vi "CLD 8 CSV file commands utility Exercise.vi"(8 "Error In":errorcluster) -> (0 "Error Out":errorcluster, 3 "Commands Out Array":T1[](array[typedef]))   [LabVIEW 2018]
doc: "CLD 8 exercise"
uses:
  CLD 8 Data Cluster.ctl
  <vilib>/Utility/file.llb/Read Delimited Spreadsheet (string).vi
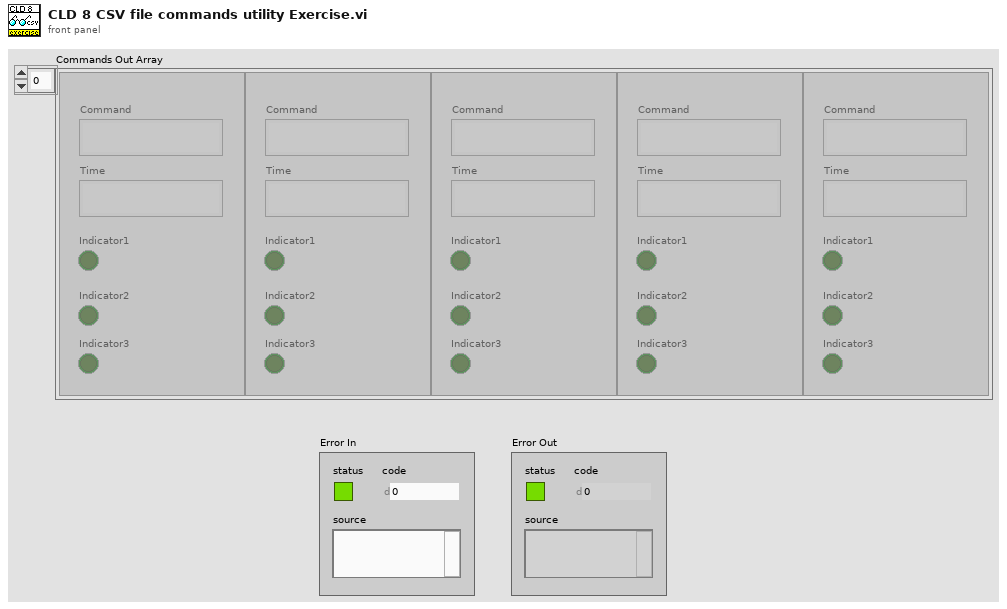
[diagram p1: front panel]
types:
  T1 = typedef "CLD 8 Data Cluster.ctl" = cluster{"Command":string, "Time":string, "Indicator1":bool, "Indicator2":bool, "Indicator3":bool}
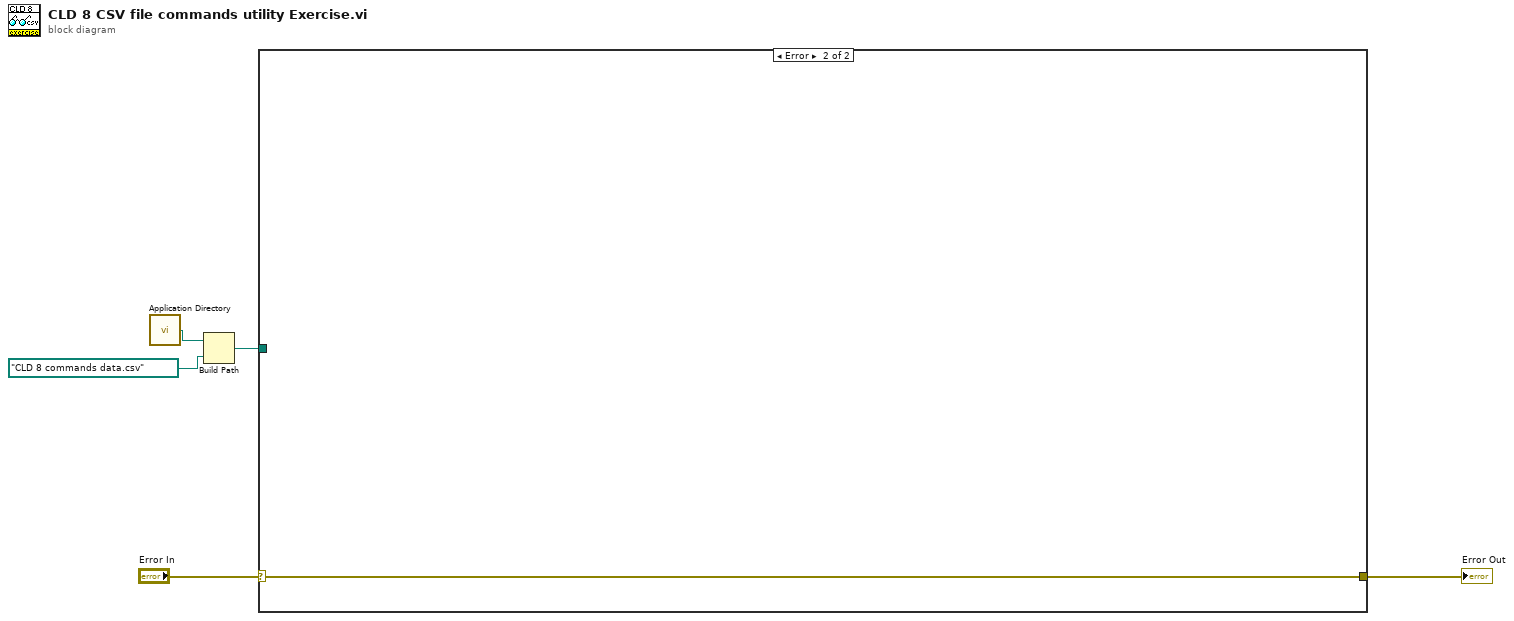
[diagram p0: block diagram]
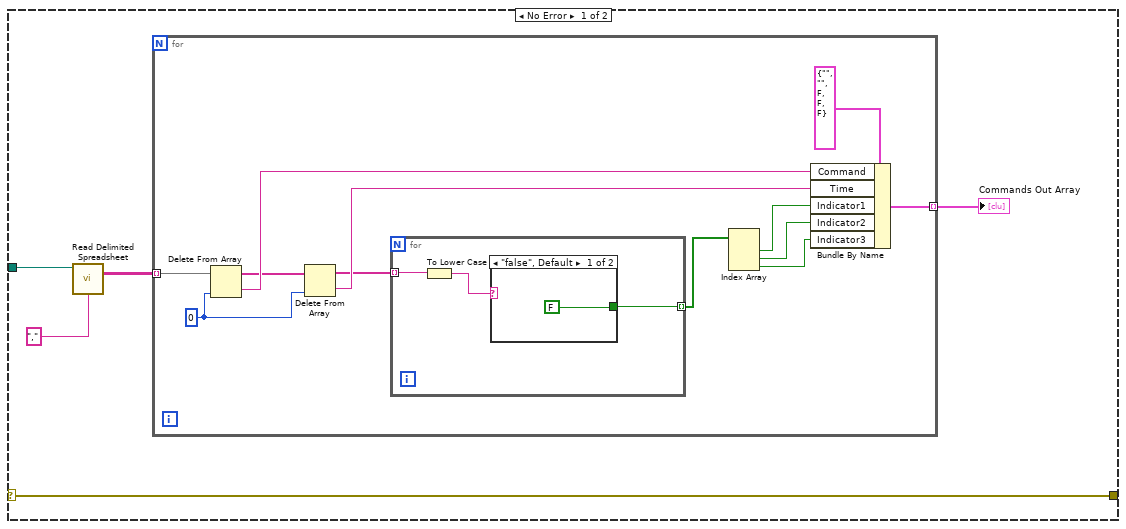
[diagram p2: hidden frame]
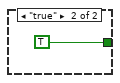
[diagram p3: hidden frame]
diagram:
  n1 = call <vilib>:"Application Directory.vi"() -> ("Application Directory"=w5:path)
  n2 = Build Path(base path=w5, name or relative path=path "CLD 8 commands data.csv") -> (appended path=w3:path)
  n3 = case shown="Error" "Error In" {
    selector: "Error In" -> [w6 w28]
    tunnel: w3 -> [w10 _]
    tunnel: [w6 w28] -> w1
    frame No Error {
      n4 = call-poly <vilib>:"Read Delimited Spreadsheet.vi"("file path (dialog if empty)"=w10, "delimiter (\\t)"="," ("delimiter (\\t)")) -> ("all rows"=w8:string[][])  [unwired: 8 in, 5 out]
      n5 = for {
        tunnel: w8 -> [w20] mode=indexing
        tunnel: [w21] -> w7 mode=indexing
        w17 = 0 ("index")
        n6 = Delete From Array(array=w20, index=w17) -> (deleted portion=w19:string, array with subset deleted=w18:string[])  [unwired: 1 in]
        n7 = Delete From Array(array=w18, index=w17) -> (deleted portion=w16:string, array with subset deleted=w15:string[])  [unwired: 1 in]
        n8 = for {
          tunnel: w15 -> [w25] mode=indexing
          tunnel: [w23] -> w14 mode=indexing
          n9 = To Lower Case(string=w25) -> (all lower case string=w24:string)
          n10 = case shown="\"false\", Default" w24 {
            tunnel: [FALSE TRUE] -> w23
            frame "false", Default {
            }
            frame "true" {
            }
          }
        }
        n11 = Index Array(array=w14) -> (element #1=w13:bool, element #2=w12:bool, element #3=w11:bool)  [unwired: 3 in]
        n12 = Bundle By Name(cluster=T1 {"Command"="", "Time"="", "Indicator1"=FALSE, "Indicator2"=FALSE, "Indicator3"=FALSE} ("Cluster"), "Command"=w19, "Time"=w16, "Indicator1"=w13, "Indicator2"=w12, "Indicator3"=w11) -> (w21:T1)
      }
      "Commands Out Array" <- w7
    }
    frame Error {
    }
  }
  "Error Out" <- w1
